vi "IV hysteresis w variable sweep rate V2.vi"() -> ()   [LabVIEW 2014]
uses:
  Environmental Chamber LabVIEW and Instruments/Drivers and Software/LabVIEW 8.2 Drivers/keithley_24xx/Keithley 24XX/Public/Data/Read (Single Point).vi
  <vilib>/Utility/file.llb/Write To Spreadsheet File (string).vi
  Environmental Chamber LabVIEW and Instruments/Drivers and Software/keithley_24xx/Keithley 24XX/Keithley 24XX.lvlib
panel:
  in  "Point delay (s)":dbl[](array[numeric])
  out "sweep points (V)":dbl[](array[numeric])
  out "Bias (V)":dbl
  out "Runtime (min)":dbl
  out "Point delay (mV/s)":dbl[](array[numeric])
  in  "RUN":bool
  out "Delay (mV/s)":dbl
  in  "voltage settings":cluster{"Vi (V)":dbl, "Vf (V)":dbl, "steps":dbl}={"Vi (V)"=-0.15, "Vf (V)"=0.15, "steps"=30.0}
  out "File path":path
  out "2420 IV curve":cluster{"X":dbl[], "Y":dbl[]}[](graph)
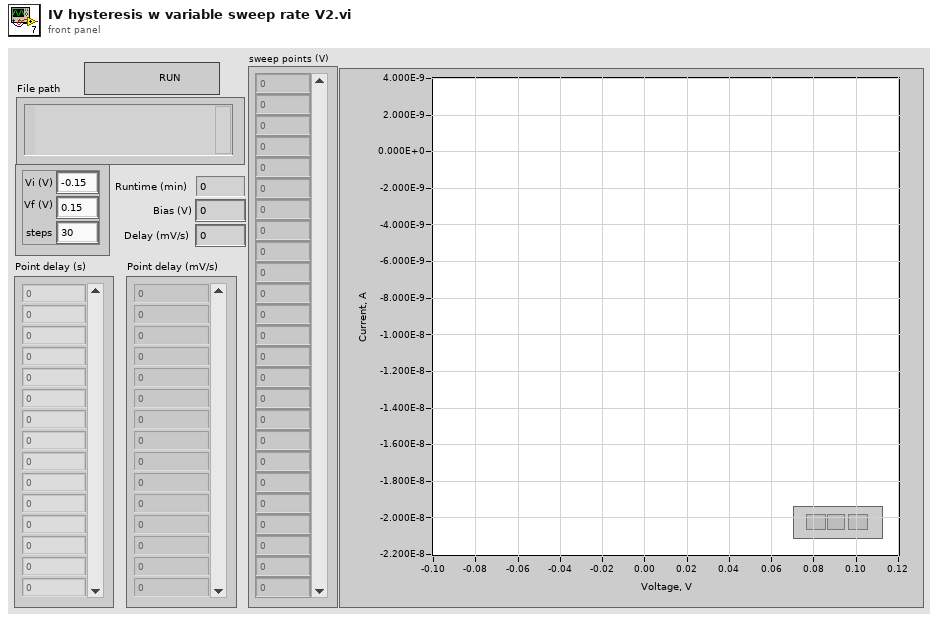
[diagram p1: front panel]
types:
  T1 = enum16{"open", "open or create", "create or replace", "create", "open (read only)"}
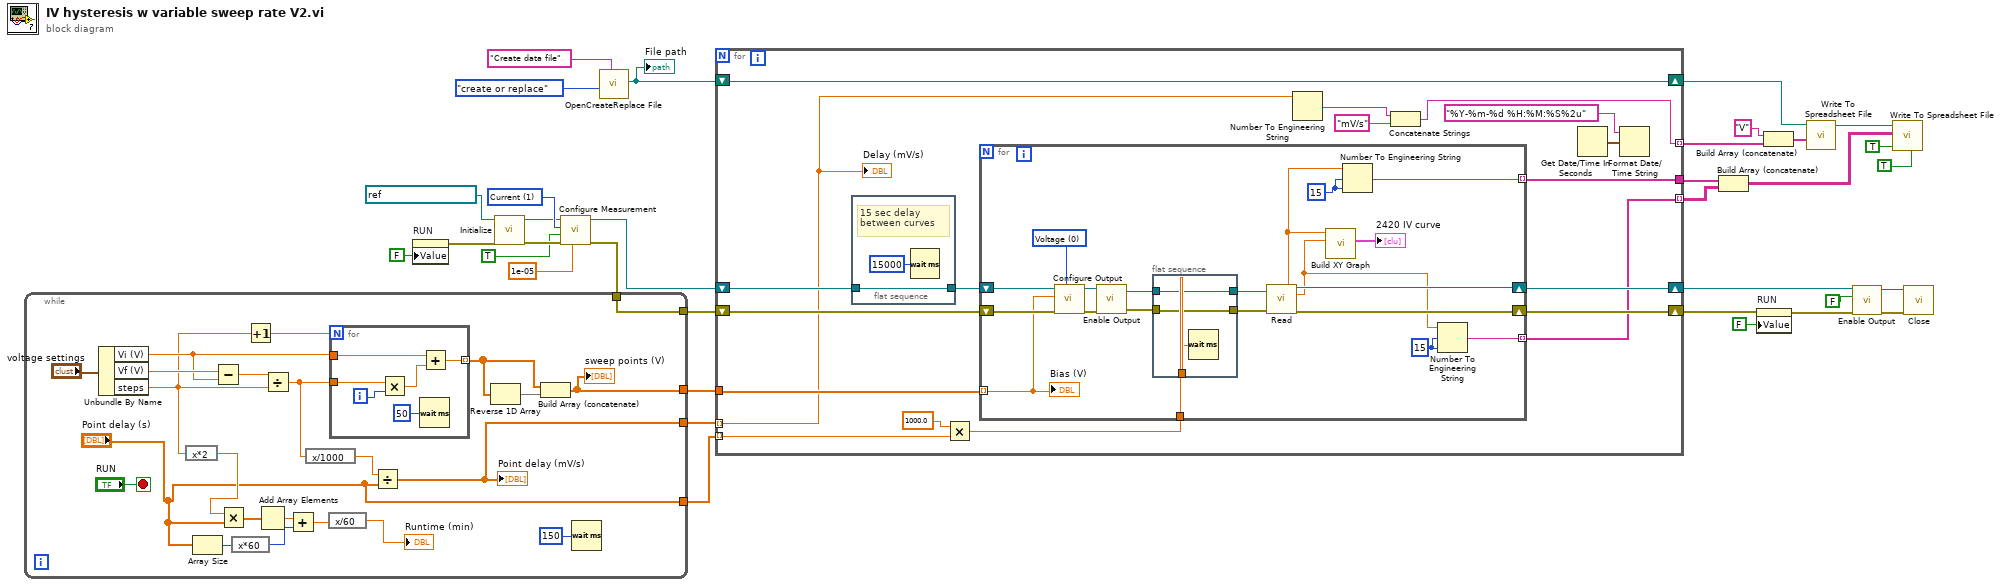
[diagram p0: block diagram]
diagram:
  w10 = u16 1 items=["Volts", "Current", "Resistance"] ("Function (0: Volts)")
  n1 = property on="RUN" class="Bool (strict)"("Value"=FALSE ("RUN")) -> (error out=w4:errorcluster)  [unwired: 2 in, 1 out]
  n2 = call "Initialize.vi"("error in (no error)"=w4, "VISA resource name"=refnum<visa-resource-name> "GPIB1::24::INSTR") -> ("error out"=w8:errorcluster, "VISA resource name out"=w9:refnum<visa-resource-name>)  [unwired: 8 in]
  n3 = call "Configure Measurement.vi"("Manual Range (1.0)"=1e-05, "error in (no error)"=w8, "Enable Auto Range (T:Enable)"=TRUE, "Function (0: Volts)"=w10, "VISA resource name"=w9) -> ("error out"=w3:errorcluster, "VISA resource name out"=w28:refnum<visa-resource-name>)  [unwired: 5 in]
  n4 = while {
    tunnel: [w53] -> w34
    tunnel: [w39] -> w33
    tunnel: w3 -> [w36]
    tunnel: [w36] -> w2
    tunnel: ["Point delay (s)"] -> w1
    stop <- "RUN" stop-if-true
    n5 = Unbundle By Name("voltage settings") -> ("Vi (V)"=w43:dbl, "Vf (V)"=w54:dbl, "steps"=w38:dbl)
    n6 = expression code="x*2"(w38) -> (w37:dbl)
    n7 = Array Size(array="Point delay (s)") -> (size(s)=w48:i32)
    n8 = Subtract(x=w54, y=w43) -> (x-y=w45:dbl)
    n9 = Multiply(x=w37, y="Point delay (s)") -> (x*y=w52:dbl[])
    n10 = expression code="x*60"(w48) -> (w47:i32)
    n11 = Increment(x=w38) -> (x+1=w42:dbl)
    n12 = Add Array Elements(numeric array=w52) -> (sum=w51:dbl)
    n13 = Divide(x=w45, y=w38) -> (x/y=w44:dbl)
    n14 = Add(x=w51, y=w47) -> (x+y=w50:dbl)
    n15 = expression code="x/1000"(w44) -> (w46:dbl)
    n16 = expression code="x/60"(w50) -> (→"Runtime (min)":dbl)
    n17 = for {
      N: w42 -> [_]
      tunnel: w44 -> [w60]
      tunnel: w43 -> [w61]
      tunnel: [w63] -> w40 mode=indexing
      i -> [w59]
      n18 = Multiply(x=w60, y=w59) -> (x*y=w62:dbl)
      n19 = Wait (ms)(milliseconds to wait=u32 50) -> ()  [unwired: 1 out]
      n20 = Add(x=w61, y=w62) -> (x+y=w63:dbl)
    }
    n21 = Divide(x=w46, y="Point delay (s)") -> (x/y=w53:dbl[])
    "Point delay (mV/s)" <- w53
    n22 = Reverse 1D Array(array=w40) -> (reversed array=w41:dbl[])
    n23 = Build Array (concatenate)(w40, w41) -> (w39:dbl[])
    "sweep points (V)" <- w39
    n24 = Wait (ms)(milliseconds to wait=u32 150) -> ()  [unwired: 1 out]
  }
  n25 = call "OpenCreateReplace File.vi"("prompt"="Create data file", "function (open:0)"=T1."create or replace") -> ("new file path"=w25:path)  [unwired: 6 in, 3 out]
  "File path" <- w25
  n26 = for {
    shift-right: [w80] -> w13
    shift-left: w2 -> [w79]
    shift-right: [w81] -> w29
    shift-left: w28 -> [w78]
    shift-right: [w76] -> w23
    shift-left: w25 -> [w76]
    tunnel: [w67] -> w20 mode=indexing
    tunnel: [w73] -> w18
    tunnel: [w72] -> w17 mode=indexing
    tunnel: w34 -> [w65] mode=indexing
    tunnel: w33 -> [w66]
    tunnel: w1 -> [w64] mode=indexing
    n27 = flat-sequence {
      tunnel: [w106] -> w77
      tunnel: w78 -> [w106]
      frame #0 {
        # "15 sec delay between curves"
        n28 = Wait (ms)(milliseconds to wait=u32 15000 ("value")) -> ()  [unwired: 1 out]
      }
    }
    n29 = Multiply(x=1000.0 ("Manual Range (1.0)"), y=w64) -> (x*y=w71:dbl)
    n30 = for {
      tunnel: [w94] -> w72 mode=indexing
      shift-right: [w100] -> w80
      shift-left: w79 -> [w99]
      shift-right: [w101] -> w81
      shift-left: w77 -> [w98]
      tunnel: [w89] -> w73 mode=indexing
      tunnel: w71 -> [w83]
      tunnel: w66 -> [w82] mode=indexing
      w87 = i16 15 ("precision (6)")
      w88 = i16 15 ("precision (6)")
      w95 = u16 0 items=["Voltage", "Current"] ("Source Mode  (0: Voltage)")
      n31 = call "Configure Output.vi"("Source Mode  (0: Voltage)"=w95, "error in (no error)"=w99, "Output Level (0)"=w82, "VISA resource name"=w98) -> ("error out"=w97:errorcluster, "VISA resource name out"=w96:refnum<visa-resource-name>)  [unwired: 6 in]
      n32 = call "Enable Output.vi"("error in (no error)"=w97, "VISA resource name"=w96) -> ("error out"=w90:errorcluster, "VISA resource name out"=w93:refnum<visa-resource-name>)  [unwired: 8 in]
      n33 = flat-sequence {
        tunnel: [w104] -> w92
        tunnel: w93 -> [w104]
        tunnel: w90 -> [w103]
        tunnel: [w103] -> w91
        tunnel: w83 -> [w102]
        frame #0 {
          n34 = Wait (ms)(milliseconds to wait=w102) -> ()  [unwired: 1 out]
        }
      }
      n35 = call-poly "Read.vi"("VISA resource name"=w92, "error in (no error)"=w91) -> ("Voltage"=w85:sgl, "VISA resource name out"=w101:refnum<visa-resource-name>, "Current"=w86:sgl, "error out"=w100:errorcluster)  [unwired: 7 in, 3 out]
      n36 = call "Build XY Graph"("Y Input"=w86, "X Input"=w85) -> ("XY Graph"=→"2420 IV curve":cluster{"X":dbl[], "Y":dbl[]}[])  [unwired: 8 in, 1 out]
      n37 = Number To Engineering String(2:w87, 3:w87, 4:w85) -> (0:w89:string)  [unwired: 1 in]
      n38 = Number To Engineering String(2:w88, 3:w88, 4:w86) -> (0:w94:string)  [unwired: 1 in]
      "Bias (V)" <- w82
    }
    n39 = Number To Engineering String(4:w65) -> (0:w69:string)  [unwired: 3 in]
    n40 = Concatenate Strings(w69, "mV/s" ("string")) -> (w67:string)
    n41 = Get Date/Time In Seconds() -> (seconds since 1Jan1904=w75:timestamp)
    n42 = Format Date/Time String(time format string (%c)="%Y-%m-%d %H:%M:%S%2u", seconds (now)=w75) -> ()  [unwired: 1 in, 1 out]
    "Delay (mV/s)" <- w65
  }
  n43 = Build Array (concatenate)(w18, w17) -> (w16:string[][])
  n44 = property on="RUN" class="Bool (strict)"(error in=w13, "Value"=FALSE ("RUN")) -> (error out=w12:errorcluster)  [unwired: 1 in, 1 out]
  n45 = Build Array (concatenate)("V", w20) -> (w19:string[])
  n46 = call-poly <vilib>:"Write To Spreadsheet File.vi"("1D data"=w19, "file path (dialog if empty)"=w23) -> ("new file path (Not A Path if cancelled)"=w22:path)  [unwired: 6 in]
  n47 = call "Enable Output.vi"("error in (no error)"=w12, "Enable Output (T: Enable)"=FALSE, "VISA resource name"=w29) -> ("error out"=w30:errorcluster, "VISA resource name out"=w32:refnum<visa-resource-name>)  [unwired: 7 in]
  n48 = call-poly <vilib>:"Write To Spreadsheet File.vi"("transpose? (no:F)"=TRUE, "append to file? (new file:F)"=TRUE ("transpose? (no:F)"), "2D data"=w16, "file path (dialog if empty)"=w22) -> ()  [unwired: 4 in, 1 out]
  n49 = call "Close.vi"("error in (no error)"=w30, "VISA resource name"=w32) -> ()  [unwired: 9 in, 1 out]
